vi "VendingMachine.vi"(1 "Item Selection":T1) -> ()   [LabVIEW 2020]
uses:
  stati.ctl
panel:
  out "RESTO":dbl
  out "PRODOTTO_EROGATO":string="CAFFE'"
  in  "Money":T2
  out "SOMMA":dbl
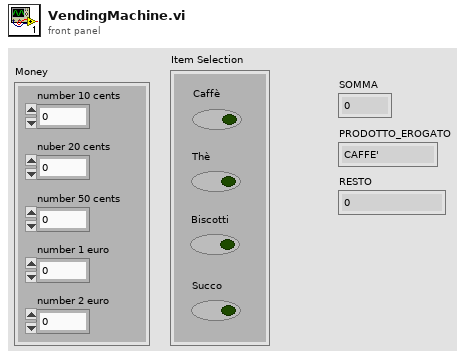
[diagram p1: front panel]
types:
  T1 = cluster{"Caffè":bool, "Thè":bool, "Biscotti":bool, "Succo":bool}
  T2 = cluster{"number 10 cents":dbl, "nuber 20 cents":dbl, "number 50 cents":dbl, "number 1 euro":dbl, "number 2 euro":dbl}
  T3 = typedef "stati.ctl" = u16
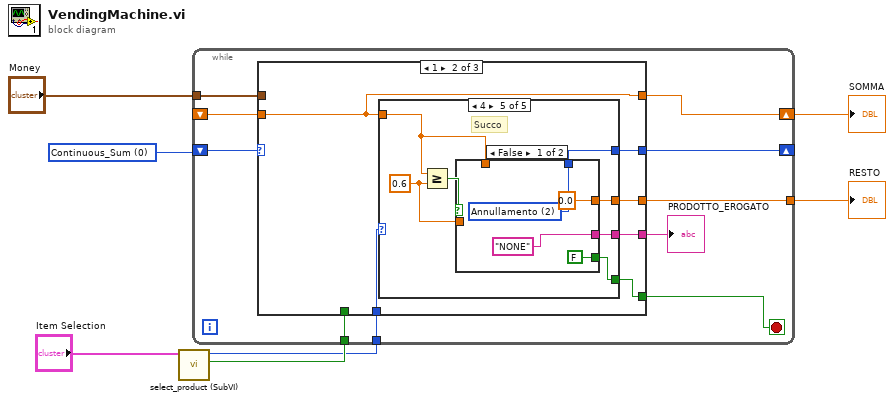
[diagram p0: block diagram]
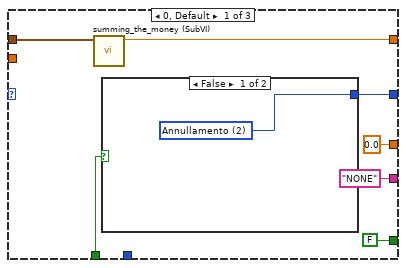
[diagram p2: hidden frame]
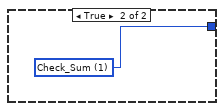
[diagram p3: hidden frame]
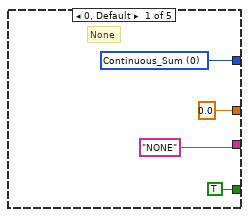
[diagram p4: hidden frame]
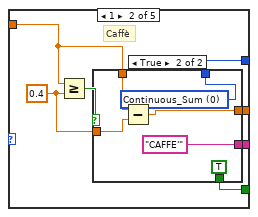
[diagram p5: hidden frame]
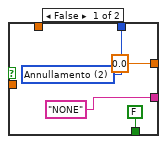
[diagram p6: hidden frame]
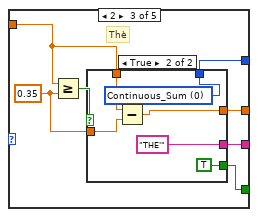
[diagram p7: hidden frame]
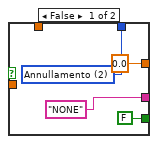
[diagram p8: hidden frame]
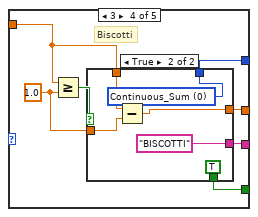
[diagram p9: hidden frame]
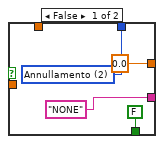
[diagram p10: hidden frame]
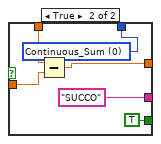
[diagram p11: hidden frame]
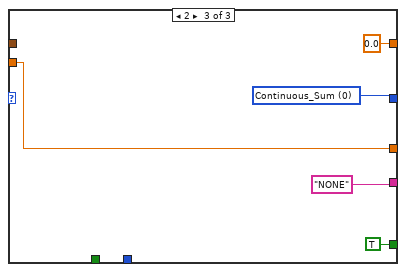
[diagram p12: hidden frame]
diagram:
  w2 = T3 0 items=["Continuous_Sum", "Check_Sum", "Annullamento"]
  n1 = call "select_product (SubVI).vi"("Item Selection"="Item Selection") -> ("Boolean"=w5:bool, "Numeric"=w3:u16)  [unwired: 9 in]
  n2 = while {
    shift-right: [w11] -> _
    shift-left: w2 -> [w12]
    tunnel: w5 -> [w16]
    tunnel: "Money" -> [w17]
    shift-right: [w15] -> w4
    shift-left: _ -> [w13]
    tunnel: w3 -> [w14]
    tunnel: [w9] -> w1
    stop <- w8 stop-if-true
    n3 = case shown="1" w12 {
      tunnel: w17 -> [w24 _ _]
      tunnel: [w23 w28 0.0 ("Numeric")] -> w15
      tunnel: w16 -> [w22 _ _]
      tunnel: w14 -> [_ w32 _]
      tunnel: w13 -> [_ w28 w109]
      tunnel: [w21 w31 w107] -> w11
      tunnel: ["NONE" w30 "NONE"] -> w10
      tunnel: [0.0 ("Numeric") w29 w109] -> w9
      tunnel: [FALSE w27 TRUE] -> w8
      frame 0, Default {
        n4 = call "summing_the_money (SubVI).vi"("Money"=w24) -> ("Numeric"=w23:dbl)  [unwired: 10 in]
        n5 = case shown="False" w22 {
          tunnel: [w25 w26] -> w21
          frame False {
            w25 = T3 2 items=["Continuous_Sum", "Check_Sum", "Annullamento"] ("Ring")
          }
          frame True {
            w26 = T3 1 items=["Continuous_Sum", "Check_Sum", "Annullamento"] ("Ring")
          }
        }
      }
      frame 1 {
        n6 = case shown="4" w32 {
          tunnel: w28 -> [_ w40 w57 w75 w92]
          tunnel: [w34 w42 w55 w74 w89] -> w31
          tunnel: ["NONE" w41 w58 w72 w91] -> w30
          tunnel: [0.0 w38 w56 w73 w90] -> w29
          tunnel: [TRUE w37 w54 w71 w88] -> w27
          frame 0, Default {
            w34 = T3 0 items=["Continuous_Sum", "Check_Sum", "Annullamento"] ("Ring")
            # "None"
          }
          frame 1 {
            w39 = 0.4 ("y")
            # "Caffè"
            n7 = Greater Or Equal?(x=w40, y=w39) -> (x >= y?=w43:bool)
            n8 = case shown="True" w43 {
              tunnel: [w47 w49] -> w42
              tunnel: ["NONE" "CAFFE'"] -> w41
              tunnel: w40 -> [_ w52]
              tunnel: w39 -> [_ w51]
              tunnel: [0.0 w50] -> w38
              tunnel: [FALSE TRUE] -> w37
              frame False {
                w47 = T3 2 items=["Continuous_Sum", "Check_Sum", "Annullamento"] ("Ring")
              }
              frame True {
                w49 = T3 0 items=["Continuous_Sum", "Check_Sum", "Annullamento"] ("Ring")
                n9 = Subtract(x=w52, y=w51) -> (x-y=w50:dbl)
              }
            }
          }
          frame 2 {
            w59 = 0.35 ("y")
            # "Thè"
            n10 = Greater Or Equal?(x=w57, y=w59) -> (x >= y?=w60:bool)
            n11 = case shown="True" w60 {
              tunnel: [w64 w66] -> w55
              tunnel: ["NONE" "THE'"] -> w58
              tunnel: w57 -> [_ w69]
              tunnel: w59 -> [_ w68]
              tunnel: [0.0 w67] -> w56
              tunnel: [FALSE TRUE] -> w54
              frame False {
                w64 = T3 2 items=["Continuous_Sum", "Check_Sum", "Annullamento"] ("Ring")
              }
              frame True {
                w66 = T3 0 items=["Continuous_Sum", "Check_Sum", "Annullamento"] ("Ring")
                n12 = Subtract(x=w69, y=w68) -> (x-y=w67:dbl)
              }
            }
          }
          frame 3 {
            w76 = 1.0 ("y")
            # "Biscotti"
            n13 = Greater Or Equal?(x=w75, y=w76) -> (x >= y?=w77:bool)
            n14 = case shown="True" w77 {
              tunnel: [w81 w83] -> w74
              tunnel: ["NONE" "BISCOTTI"] -> w72
              tunnel: w75 -> [_ w86]
              tunnel: w76 -> [_ w85]
              tunnel: [0.0 w84] -> w73
              tunnel: [FALSE TRUE] -> w71
              frame False {
                w81 = T3 2 items=["Continuous_Sum", "Check_Sum", "Annullamento"] ("Ring")
              }
              frame True {
                w83 = T3 0 items=["Continuous_Sum", "Check_Sum", "Annullamento"] ("Ring")
                n15 = Subtract(x=w86, y=w85) -> (x-y=w84:dbl)
              }
            }
          }
          frame 4 {
            w93 = 0.6 ("y")
            # "Succo"
            n16 = Greater Or Equal?(x=w92, y=w93) -> (x >= y?=w94:bool)
            n17 = case shown="False" w94 {
              tunnel: [w98 w100] -> w89
              tunnel: ["NONE" "SUCCO"] -> w91
              tunnel: w92 -> [_ w103]
              tunnel: w93 -> [_ w102]
              tunnel: [0.0 w101] -> w90
              tunnel: [FALSE TRUE] -> w88
              frame False {
                w98 = T3 2 items=["Continuous_Sum", "Check_Sum", "Annullamento"] ("Ring")
              }
              frame True {
                w100 = T3 0 items=["Continuous_Sum", "Check_Sum", "Annullamento"] ("Ring")
                n18 = Subtract(x=w103, y=w102) -> (x-y=w101:dbl)
              }
            }
          }
        }
      }
      frame 2 {
        w107 = T3 0 items=["Continuous_Sum", "Check_Sum", "Annullamento"] ("Ring")
      }
    }
    "PRODOTTO_EROGATO" <- w10
  }
  "SOMMA" <- w4
  "RESTO" <- w1
